vi "Create Ack.vi"(6 "sample rate":dbl=1000.0 format="%#_6p", 7 "OVS":u8=16, 8 "error in (no error)":errorcluster) -> (0 "error out":errorcluster, 3 "Digital Waveform Graph":digitalwaveform(graph))   [LabVIEW 2013]
uses:
  <vilib>/Waveform/DWDTOps.llb/Digital Pattern Generator (Single Value).vi
  <vilib>/Waveform/DWDTOps.llb/DWDT Append Digital Samples.vi
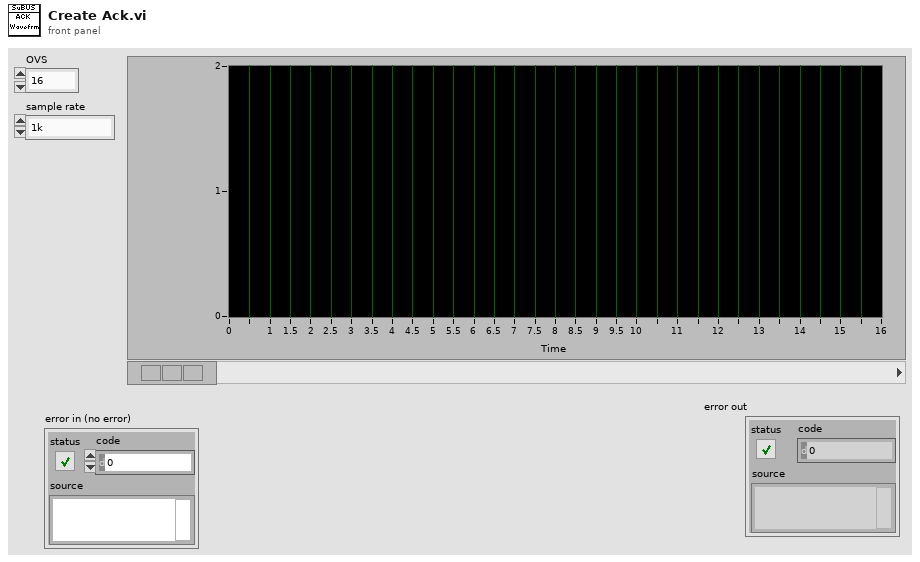
[diagram p1: front panel]
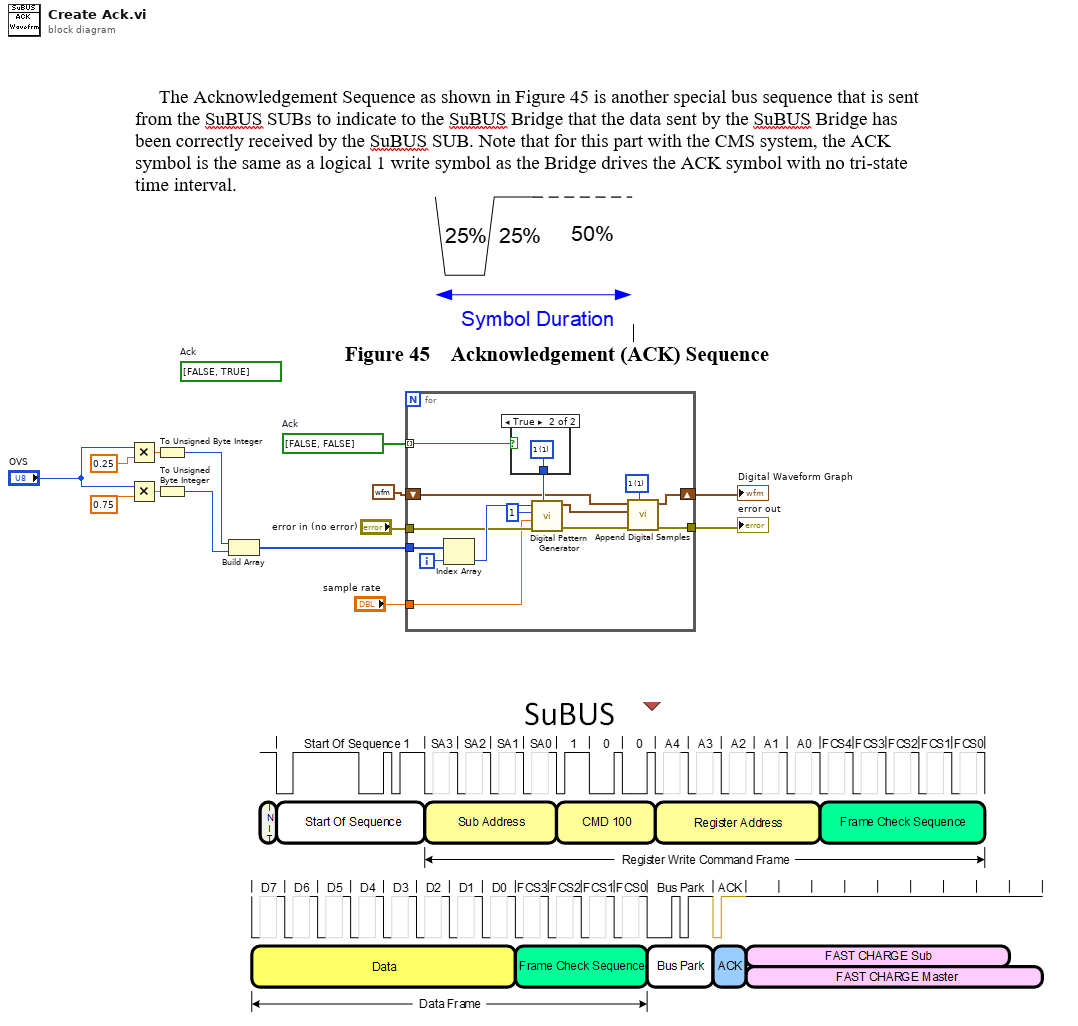
[diagram p0: block diagram]
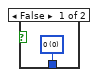
[diagram p2: hidden frame]
diagram:
  (unwired) bool[] [FALSE, TRUE]  # Ack
  w7 = bool[] [FALSE, FALSE]  # Ack
  n1 = Multiply(x="OVS", y=0.25) -> (x*y=w14:dbl)
  n2 = Multiply(x="OVS", y=0.75) -> (x*y=w12:dbl)
  n3 = To Unsigned Byte Integer(number=w14) -> (unsigned 8bit integer=w10:u8)
  n4 = To Unsigned Byte Integer(number=w12) -> (unsigned 8bit integer=w9:u8)
  n5 = Build Array(w10, w9) -> (w8:u8[])
  n6 = for {
    tunnel: w8 -> [w28]
    tunnel: w7 -> [w25] mode=indexing
    shift-right: [w19] -> w2
    shift-left: digitalwaveform {"t0"=timestamp(0 s since 1904-01-01), "dt"=0.0, "Y"={"transitions"=[], "data"=[]}} ("digital waveform out") -> [w18]
    tunnel: "error in (no error)" -> [w17]
    tunnel: [w16] -> w3
    tunnel: "sample rate" -> [w15]
    i -> [w27]
    w22 = u8 1 items=["0", "1", "Z", "L", "H", "X", "T", "V"] ("default value")
    n7 = Index Array(array=w28, index=w27) -> (element=w23:u8)
    n8 = case shown="True" w25 {
      tunnel: [w29 w30] -> w24
      frame False {
        w29 = u8 0 items=["0", "1", "Z", "L", "H", "X", "T", "V"] ("value")
      }
      frame True {
        w30 = u8 1 items=["0", "1", "Z", "L", "H", "X", "T", "V"] ("value")
      }
    }
    n9 = call-poly <vilib>:"Digital Pattern Generator.vi"("value"=w24, "error in (no error)"=w17, "sample rate"=w15, "number of signals"=u32 1, "number of samples"=w23) -> ("error out"=w21:errorcluster, "digital waveform"=w20:digitalwaveform)  [unwired: 5 in]
    n10 = call-poly <vilib>:"Append Digital Samples.vi"("default value"=w22, "error in (no error)"=w21, "digital waveform B"=w20, "digital waveform A"=w18) -> ("error out"=w16:errorcluster, "digital waveform out"=w19:digitalwaveform)  [unwired: 6 in]
  }
  "error out" <- w3
  "Digital Waveform Graph" <- w2
